vi "Vertical Fill Slide (Silver).vi"() -> ()   [LabVIEW 2012]
panel:
  in  "Vertical Fill Slide":dbl(slide) scale=0.0..10.0
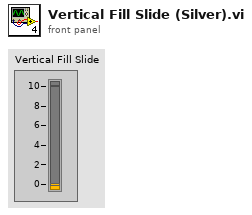
[diagram p1: front panel]
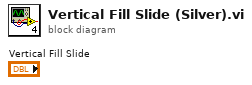
[diagram p0: block diagram]
diagram:
